vi "testFlushTelQueueToDds.vi"(8 "error in (no error)":errorcluster) -> (0 "error out":errorcluster)   [LabVIEW 2018]
doc: "Test the flushTelQueue.vi with queueToDds option."
uses:
  src/TcpServer/TcpServer.lvclass
  src/TcpServer/TcpServer.lvclass/TcpServer.ctl
  src/TcpServerBase/TcpServerBase.lvclass/TcpServerBase.ctl
  src/TcpServerTel/TcpServerTel.lvclass
  home/pcortes/github/ts_labview_tcp_json/src/TcpServerBase/TcpServerBase.lvclass
  <vilib>/addons/_JKI Toolkits/Caraya/classes/Assert/Assert Equal Value_Variant.vi
  <vilib>/addons/_JKI Toolkits/Caraya/classes/Test/Test.lvclass
  <vilib>/addons/_JKI Toolkits/Caraya/classes/Assert/Assert.lvclass
  src/TcpServerBase/TcpServerBase.lvclass
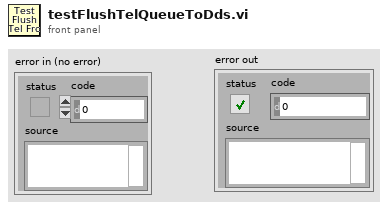
[diagram p1: front panel]
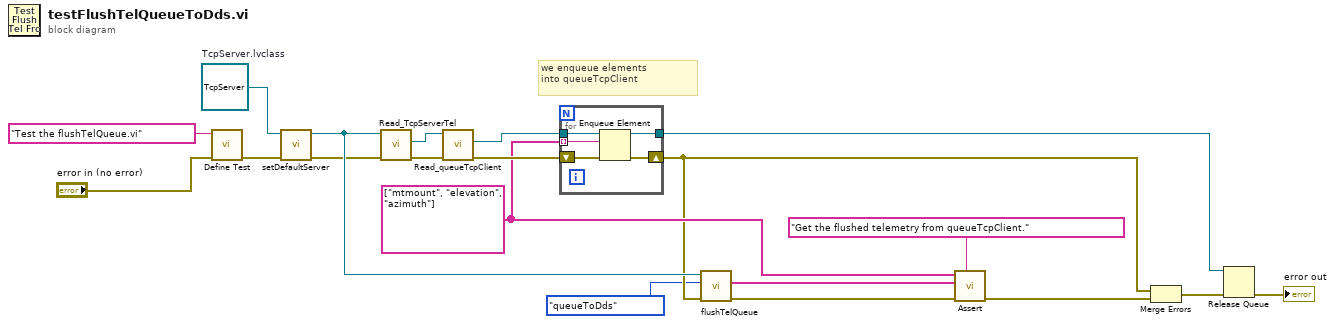
[diagram p0: block diagram]
diagram:
  w3 = string[] ["mtmount", "elevation", "azimuth"]
  w17 = refnum<class "TcpServer.lvclass"> refnum  # TcpServer.lvclass
  # "we enqueue elements\ninto queueTcpClient"
  n1 = call <vilib>:"Define Test.vi"("error in (no error)"="error in (no error)", "Label (VI Title)"="Test the flushTelQueue.vi") -> ("error out"=w19:errorcluster)  [unwired: 9 in]
  n2 = call "setDefaultServer.vi"("error in (no error)"=w19, "TcpServer.lvclass"=w17) -> ("error out"=w6:errorcluster, "tcpServer out"=w7:refnum<class "TcpServer.lvclass">)  [unwired: 8 in]
  n3 = call "Read_TcpServerTel.vi"("error in (no error)"=w6, "TcpServer in"=w7) -> ("error out"=w13:errorcluster, "TcpServerTel.lvclass"=w14:refnum<class "TcpServerTel.lvclass">)  [unwired: 7 in, 1 out]
  n4 = call "Read_queueTcpClient.vi"("error in (no error)"=w13, "TcpServerBase in"=w14) -> ("error out"=w10:errorcluster, "queueTcpClient"=w9:refnum<queue>)  [unwired: 7 in, 1 out]
  n5 = for {
    tunnel: w9 -> [w24]
    tunnel: w3 -> [w23] mode=indexing
    tunnel: [w21] -> w8
    shift-right: [w22] -> w2
    shift-left: w10 -> [w25]
    n6 = Enqueue Element(queue=w24, element=w23, error in (no error)=w25) -> (queue out=w21:refnum<queue>, error out=w22:errorcluster)  [unwired: 1 in, 1 out]
  }
  n7 = call "flushTelQueue.vi"("error in (no error)"=w2, "queueName"=enum16{"queueFromDds", "queueToDds"}."queueToDds", "TcpServer in"=w7) -> ("error out"=w5:errorcluster, "telemetry flushed"=w4:string[])  [unwired: 6 in, 1 out]
  n8 = call-poly <vilib>:"Assert.vi"("Label"="Get the flushed telemetry from queueTcpClient.", "error in (no error)"=w5, "Y"=w4, "X"=w3) -> ("error out"=w15:errorcluster)  [unwired: 7 in]
  n9 = Merge Errors(w2, w15) -> (w11:errorcluster)
  n10 = Release Queue(queue=w8, error in (no error)=w11) -> (error out=→"error out":errorcluster)  [unwired: 1 in, 2 out]
